vi "Configure Dialog.vi"(8 "error in (no error)":errorcluster, 11 "Configure Alarms Msg.lvclass":refnum<class "Configure Alarms Msg.lvclass">) -> (0 "error out":errorcluster, 2 "Ok?":bool, 3 "Configure Alarms Msg.lvclass":refnum<class "Configure Alarms Msg.lvclass">)   [LabVIEW 2015, in "LS218.lvlib" / "Configure Alarms Msg.lvclass"]
uses:
  Configure Alarms Msg.lvclass
  Configure Alarms Msg.lvclass/Configure Alarms Msg.ctl
panel:
  in  "Boolean Alarm Controls":T1
  in  "Alarm Limits":T2
  in  "Cancel Button":bool
  in  "OK Button":bool
  in  "Input (0)":i32
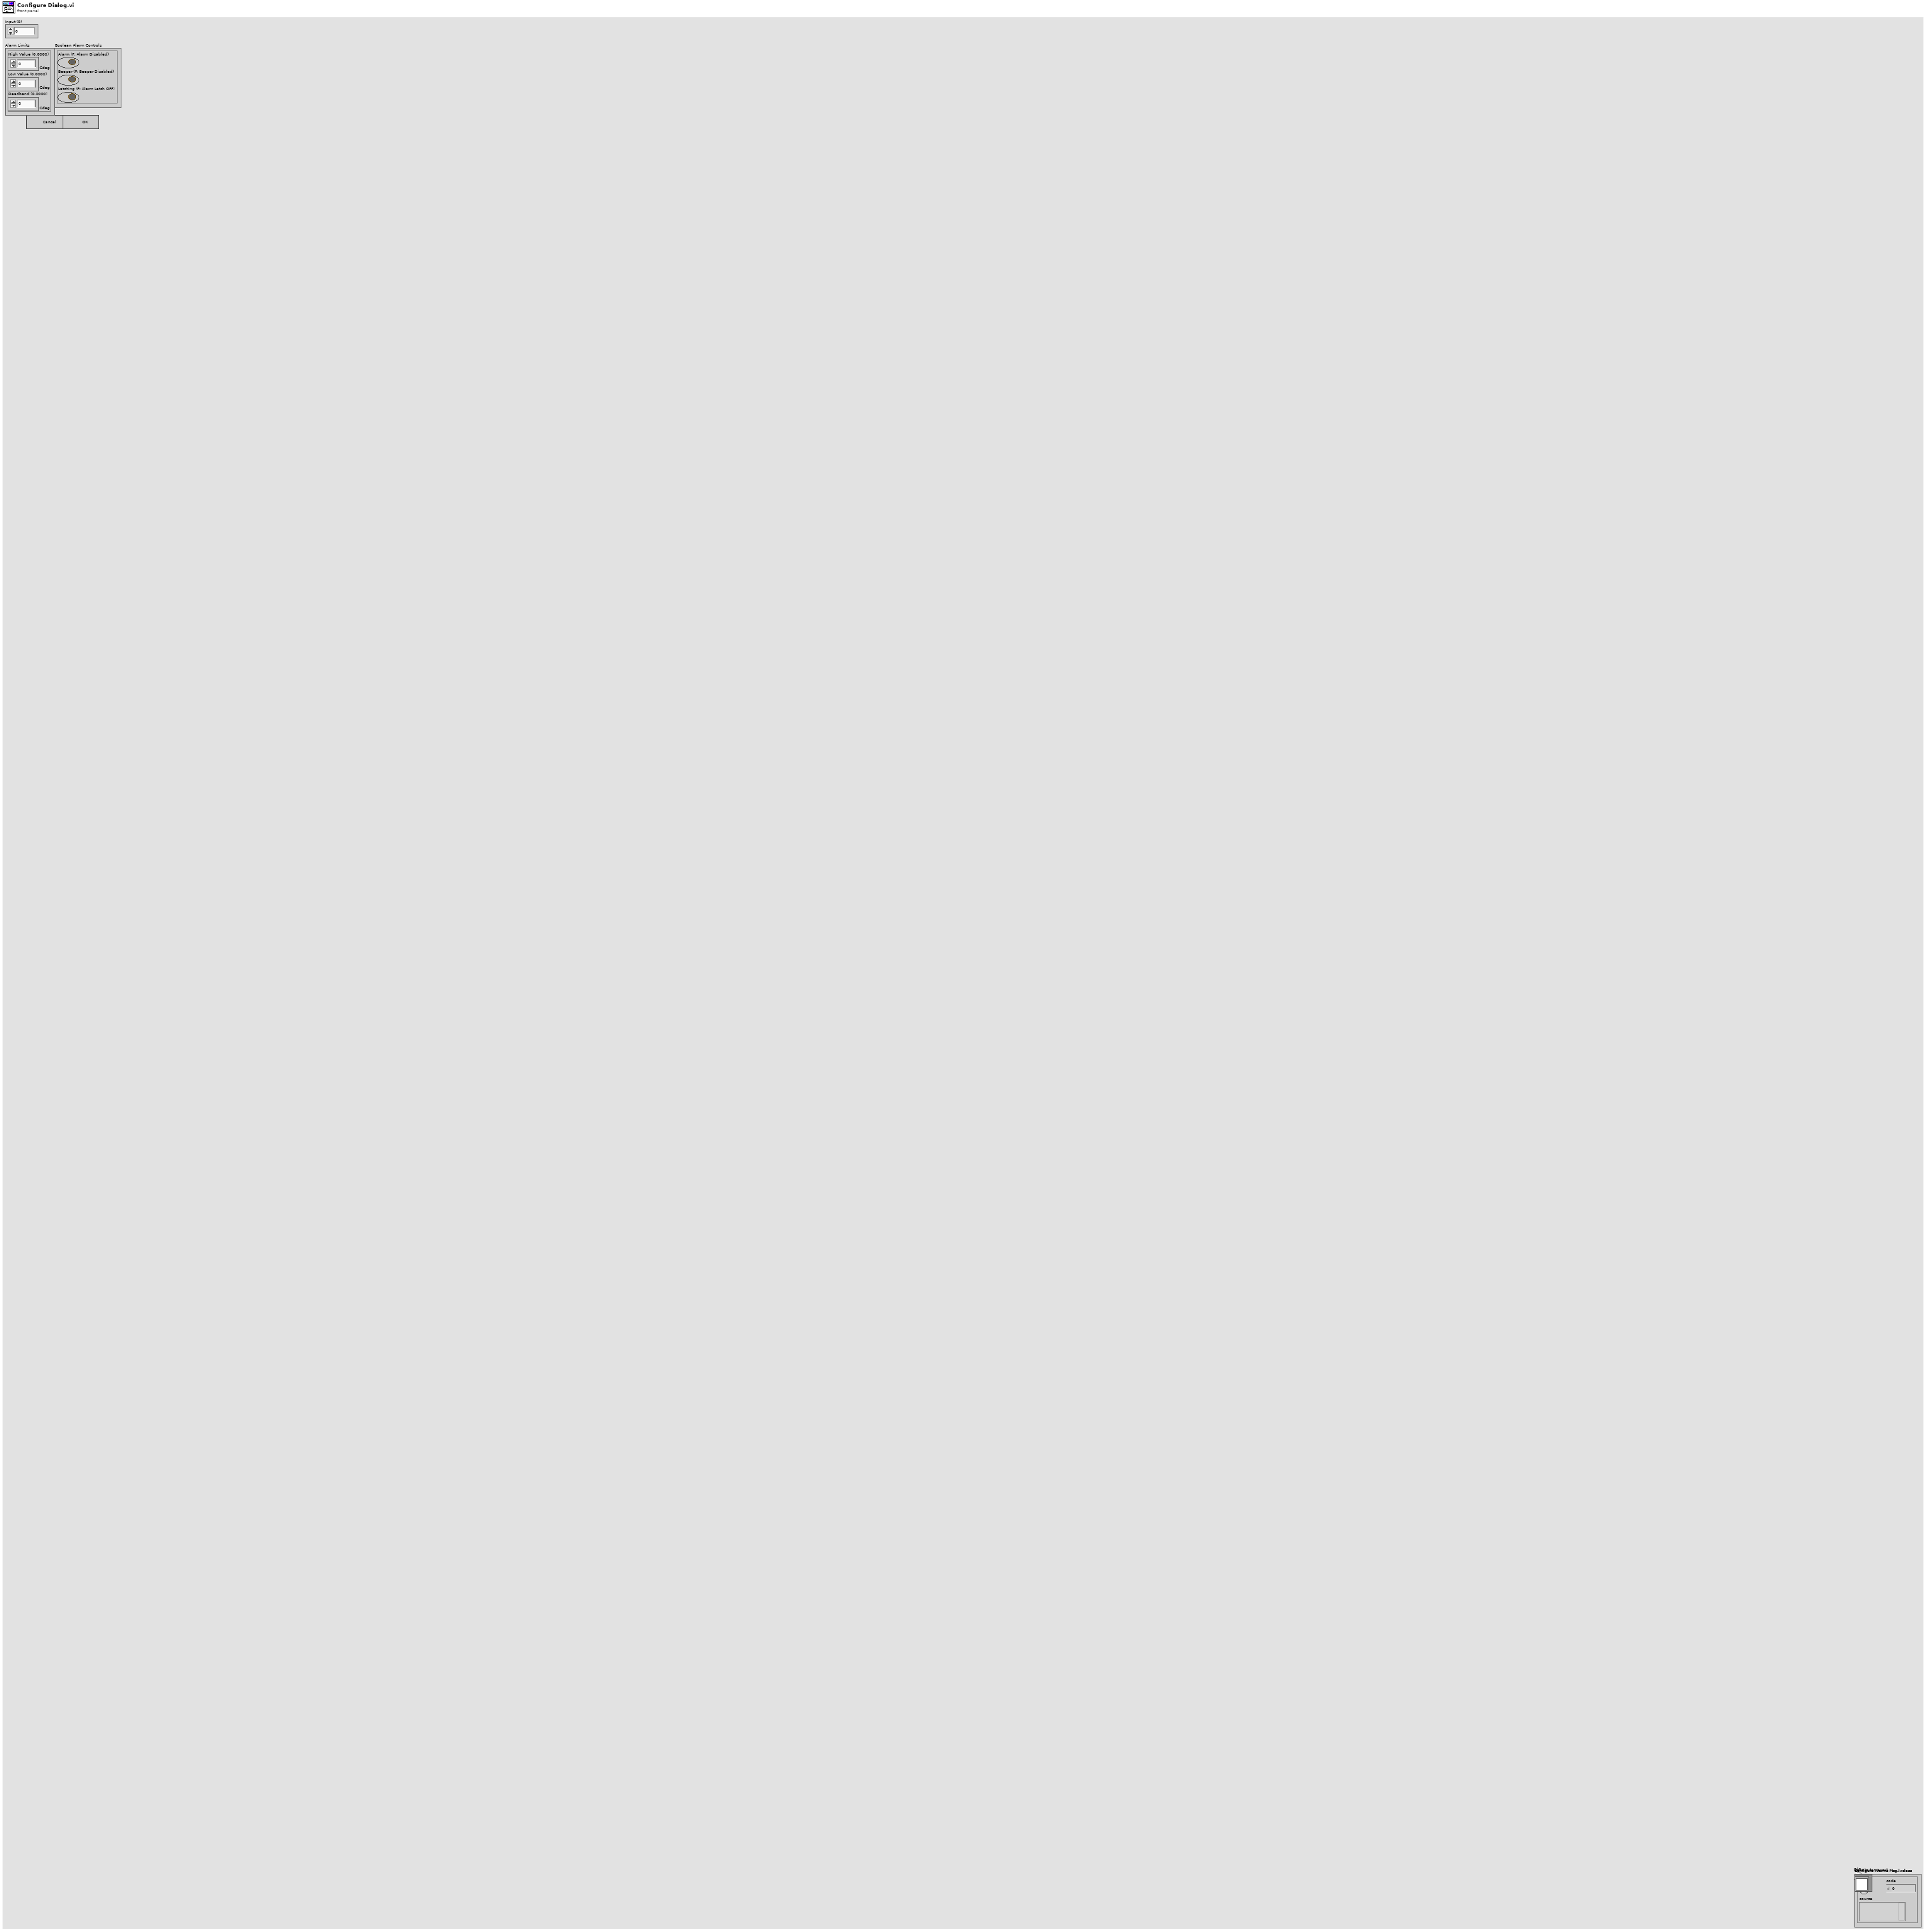
[diagram p1: front panel]
types:
  T1 = cluster{"Alarm (F: Alarm Disabled)":bool, "Beeper (F: Beeper Disabled)":bool, "Latching (F: Alarm Latch OFF)":bool}
  T2 = cluster{"High Value (0.0000)":dbl[unit], "Low Value (0.0000)":dbl[unit], "Deadband (0.0000)":dbl[unit]}
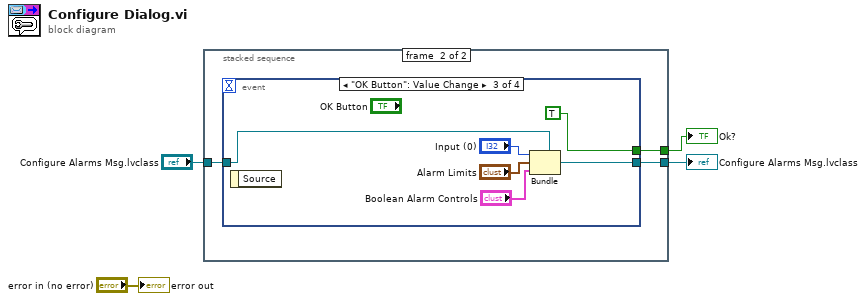
[diagram p0: block diagram]
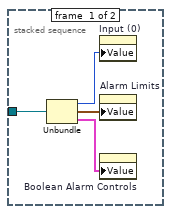
[diagram p2: hidden frame]
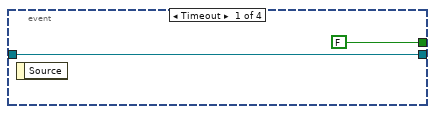
[diagram p3: hidden frame]
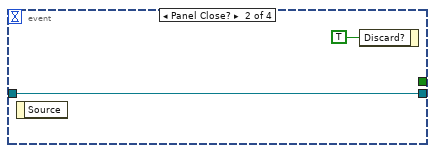
[diagram p4: hidden frame]
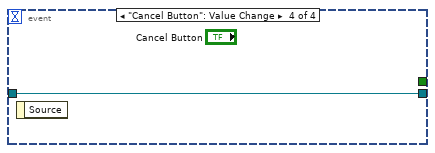
[diagram p5: hidden frame]
diagram:
  n1 = stacked-sequence {
    tunnel: [_ w11] -> w3
    tunnel: [_ w10] -> w2
    tunnel: "Configure Alarms Msg.lvclass" -> [w8 w9]
    frame #0 {
      n2 = Unbundle ("Seq0Unbundler")(w8) -> (w7:i32, w6:T2, w5:T1)
      n3 = property on="Input (0)" class="DigNum (strict)"("Value"=w7) -> ()  [unwired: 2 in, 2 out]
      n4 = property on="Alarm Limits" class="Clust (strict)"("Value"=w6) -> ()  [unwired: 2 in, 2 out]
      n5 = property on="Boolean Alarm Controls" class="Clust (strict)"("Value"=w5) -> ()  [unwired: 2 in, 2 out]
    }
    frame #1 {
      n6 = event shown="[2] \"OK Button\": Value Change" {
        selector: _ -> [_ _ _ _]
        dyn-events: _ -> [_ _ _ _]
        timeout: _ -> [_ _ _ _]
        tunnel: [w12 w14 w19 w22] -> w10
        tunnel: w9 -> [w12 w14 w21 w22]
        tunnel: [FALSE _ TRUE _] -> w11
        event Timeout {
          n7 = event-data() -> ()  [unwired: 1 in, 1 out]
        }
        event Panel Close? {
          n8 = event-data() -> ()  [unwired: 1 in, 1 out]
          n9 = event-data ("Event Filter Node")("Discard?"=TRUE) -> ()  [unwired: 1 in, 1 out]
        }
        event "OK Button": Value Change {
          n10 = event-data() -> ()  [unwired: 1 in, 1 out]
          n11 = Bundle ("Main-Bundler")(cluster=w21, "Input (0)", "Alarm Limits", "Boolean Alarm Controls") -> (w19:refnum<class "Configure Alarms Msg.lvclass">)
        }
        event "Cancel Button": Value Change {
          n12 = event-data() -> ()  [unwired: 1 in, 1 out]
        }
      }
    }
  }
  "Ok?" <- w3
  "Configure Alarms Msg.lvclass" <- w2
  "error out" <- "error in (no error)"
